vi "lab #5 (while loop using random).vi"() -> ()   [LabVIEW 2016]
panel:
  out "x 2":i32
  out "number":dbl
  in  "x":dbl
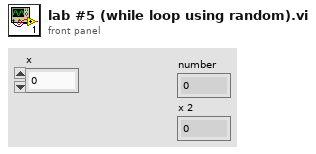
[diagram p1: front panel]
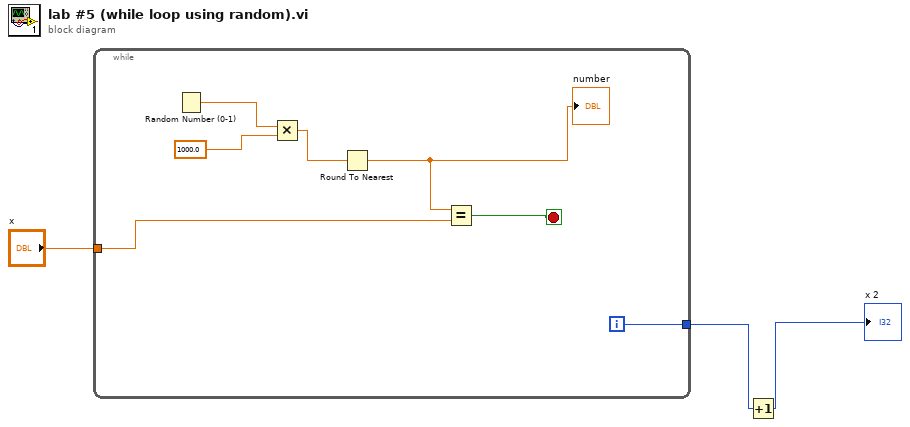
[diagram p0: block diagram]
diagram:
  n1 = while {
    tunnel: "x" -> [w6]
    tunnel: [w4] -> w2
    i -> [w4]
    stop <- w7 stop-if-true
    n2 = Random Number (0-1)() -> (number: 0 to 1=w9:dbl)
    n3 = Multiply(x=w9, y=1000.0) -> (x*y=w8:dbl)
    n4 = Round To Nearest(number=w8) -> (nearest integer value=w5:dbl)
    "number" <- w5
    n5 = Equal?(x=w5, y=w6) -> (x = y?=w7:bool)
  }
  n6 = Increment(x=w2) -> (x+1=→"x 2":i32)
